vi "Initialize.vi"(8 "error in":errorcluster, 11 "AF Trace Queue in":refnum<class "AF Trace Queue.lvclass">) -> (0 "error out":errorcluster, 3 "AF Trace Queue out":refnum<class "AF Trace Queue.lvclass">)   [LabVIEW 2020, in "AF Trace Queue.lvclass"]
uses:
  AF Trace Queue.lvclass
  AF Trace Queue.lvclass/AF Trace Queue.ctl
panel:
  out "Debug Alias":string="AFDebugTrace"
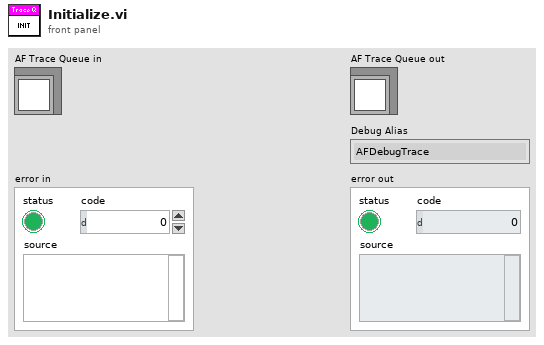
[diagram p1: front panel]
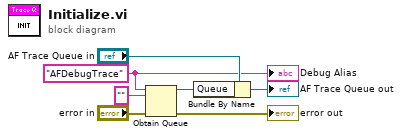
[diagram p0: block diagram]
diagram:
  w1 = "AFDebugTrace" ("Name")
  n1 = Obtain Queue(name (unnamed)=w1, element data type="", error in (no error)="error in") -> (queue out=w3:refnum<queue>, error out=→"error out":errorcluster)  [unwired: 2 in, 1 out]
  n2 = Bundle By Name(cluster="AF Trace Queue in", "Queue"=w3) -> (→"AF Trace Queue out":refnum<class "AF Trace Queue.lvclass">)
  "Debug Alias" <- w1
